vi "Plot Maximize Button Exists.vi"(8 "error in (no error)":errorcluster, 11 "BluePlotHandle in":refnum<class "RocketPlotHandle.lvclass">) -> (0 "error out":errorcluster, 2 "Plot Maximize Button exists?":bool, 3 "BluePlotHandle out":refnum<class "RocketPlotHandle.lvclass">)   [LabVIEW 2021, in "RocketPlotHandle.lvclass"]
uses:
  RocketPlotHandle.lvclass
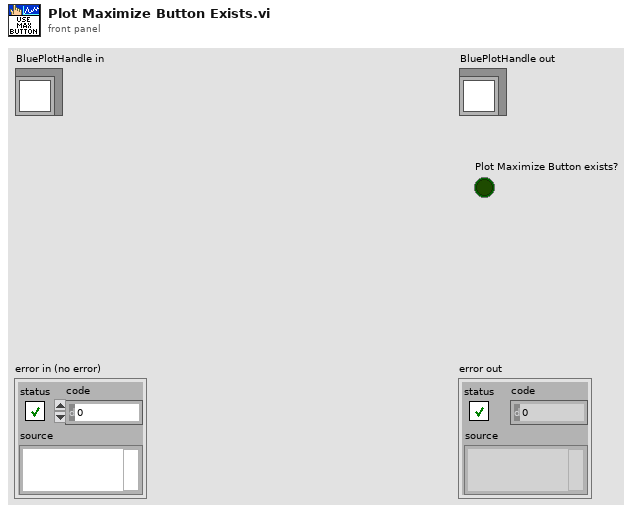
[diagram p1: front panel]
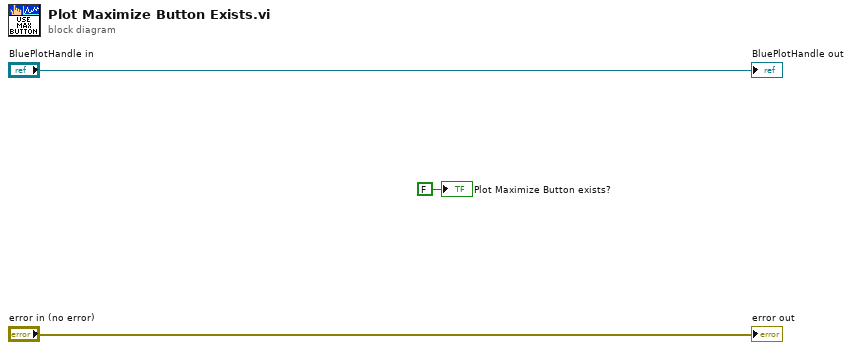
[diagram p0: block diagram]
diagram:
  "error out" <- "error in (no error)"
  "BluePlotHandle out" <- "BluePlotHandle in"
  "Plot Maximize Button exists?" <- FALSE ("Plot Maximize Button exists?")
